vi "SequencerPrototype.vi"() -> ()   [LabVIEW 2013]
uses:
  Controls/SequenceCluster.ctl
panel:
  in  "Sequence Control":string[][](table)=[["1", "A-", "AND", "B-", "AND", "", "", "S1", "SET", ""], ["1", "A+", "AND", "S1", "AND", "", "", "S2", "SET", ""], ["3", "B+", "AND", "S2", "AND", "", "", "S3", "SET", ""], ["4", "A-", "AND", "S3", "AND", "", "", "S4", "SET", ""], ["5", "B-", "AND", "S4", "AND", "", "", "S5", "SET", ""], ["6", "S1", "AND", "S3", "NOT", "AND", "A", "OUT", "", ""], ["7", "S2", "AND", "S4", "NOT", "AND", "B", "OUT", "", ""], ["8", "S5", "AND", "S1", "RES", "S2", "RES", "S3", "RES", ""], ["9", "S5", "AND", "S4", "RES", "S5", "RES", "", "", ""]]
  out "error out":errorcluster
  in  "Update Sequence":bool
  out "Inputs":string[](array[string])=["A", "A+", "A-", "B", "B+", "B-", "S1", "S2", "S3", "S4", "S5", "S6", "S7"]
  out "Outputs":string[](array[string])=["A", "A+", "A-", "B", "B+", "B-", "S1", "S2", "S3", "S4", "S5", "S6", "S7"]
  in  "Inputs":bool[](array[boolean])
  out "Outputs":bool[](array[boolean])
  in  "stop":bool
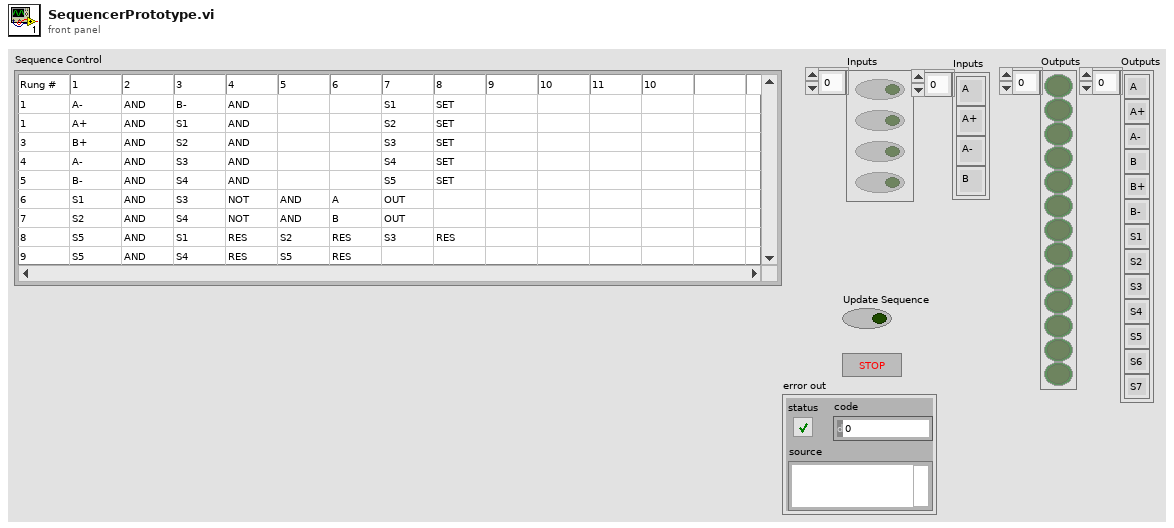
[diagram p1: front panel]
types:
  T1 = typedef "SequenceCluster.ctl" = cluster{"Sequence":string[][], "Rung Index":i32[], "Rung Lenght":i32[]}
  T2 = typedef "tag bus.lvlib/data table.lvlib/data table.ctl" = cluster{"Double":dbl[], "Single":sgl[], "I64":i64[], "I32":i32[], "I16":i16[], "I8":i8[], "U64":u64[], "U32":u32[], "U16":u16[], "U8":u8[], "Boolean":bool[], "String":string[], "Array of Double":cluster{"DBL Array":dbl[]}[], "Array of Single":cluster{"SGL Array":sgl[]}[], "Array of I64":cluster{"I64 Array":i64[]}[], "Array of I32":cluster{"I32 Array":i32[]}[], "Array of I16":cluster{"I16 Array":i16[]}[], "Array of I8":cluster{"I8 Array":i8[]}[], "Array of U64":cluster{"U64 Array":u64[]}[], "Array of U32":cluster{"U32 Array":u32[]}[], "Array of U16":cluster{"U16 Array":u16[]}[], "Array of U8":cluster{"U8 Array":u8[]}[], "Array of Boolean":cluster{"Boolean Array":bool[]}[], "Array of String":cluster{"String Array":string[]}[]}
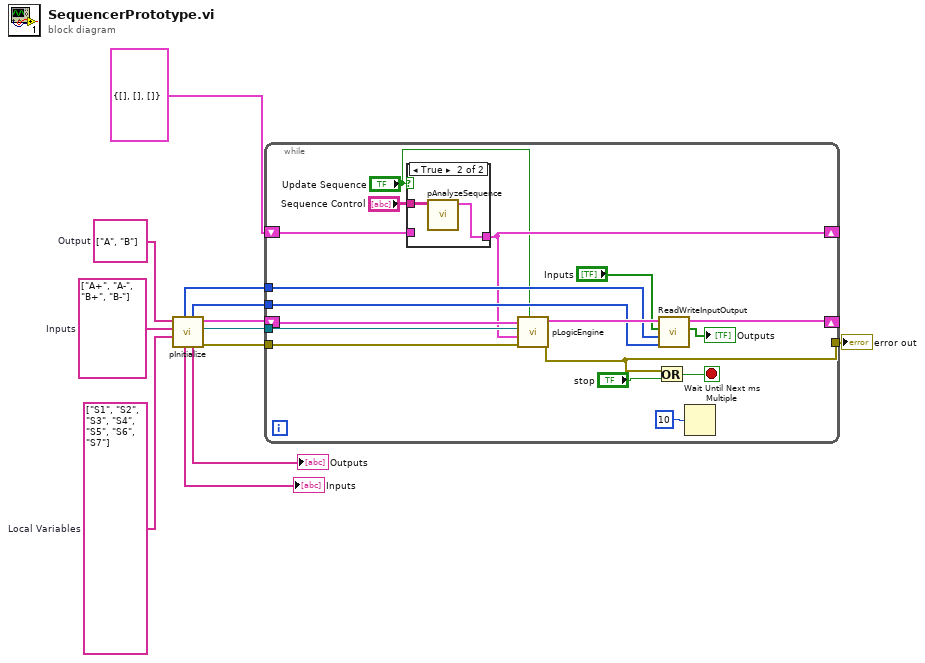
[diagram p0: block diagram]
diagram:
  w11 = string[] ["A", "B"]  # Output
  w10 = string[] ["A+", "A-", "B+", "B-"]  # Inputs
  w12 = string[] ["S1", "S2", "S3", "S4", "S5", "S6", "S7"]  # Local Variables
  n1 = call "pInitialize.vi"("Internal"=w12, "Inputs in"=w10, "Output"=w11) -> ("error out"=w6:errorcluster, "data dictionary out"=w2:refnum<class "data dictionary.lvclass">, "default data table"=w5:T2, "Outputs"=→"Outputs":string[], "Input Index"=w3:i32[], "Inputs out"=→"Inputs":string[], "Output Index"=w4:i32[])  [unwired: 2 in]
  n2 = while {
    shift-right: [w17] -> _
    shift-left: w5 -> [w19]
    shift-right: [w15] -> _
    shift-left: T1 {"Sequence"=[], "Rung Index"=[], "Rung Lenght"=[]} ("Sequence") -> [w14]
    tunnel: w6 -> [w27]
    tunnel: [w24] -> w7
    tunnel: w4 -> [w21]
    tunnel: w3 -> [w20]
    tunnel: w2 -> [w18]
    stop <- w25 stop-if-true
    n3 = case shown="True" "Update Sequence" {
      tunnel: "Sequence Control" -> [_ w32]
      tunnel: [w30 w31] -> w15
      tunnel: w14 -> [w30 _]
      frame False {
      }
      frame True {
        n4 = call "pAnalyzeSequence.vi"("Array 3"=w32) -> ("Sequence"=w31:T1)  [unwired: 10 in]
      }
    }
    n5 = call "pLogicEngine.vi"("Update"="Update Sequence", "error in"=w27, "Sequence"=w15, "data dictionary in"=w18, "default data table"=w19) -> ("error out"=w24:errorcluster, "data table out"=w23:T2)  [unwired: 5 in]
    n6 = Or(x=w24, y="stop") -> (x .or. y?=w25:bool)
    n7 = call "ReadWriteInputOutput.vi"("Input Index"=w20, "Output Index"=w21, "Inputs"="Inputs", "data table in"=w23) -> ("Outputs"=→"Outputs":bool[], "data table out"=w17:T2)  [unwired: 6 in]
    n8 = Wait Until Next ms Multiple(millisecond multiple=u32 10) -> ()  [unwired: 1 out]
  }
  "error out" <- w7
